vi "14_NOV_VARY_I_GET_V_FOR_LOOP.vi"() -> ()   [LabVIEW 2020]
uses:
  <instrlib>/Agilent B2900 Series/Agilent B2900 Series.lvlib
panel:
  out "SCPI COMMAND":string
  out "XY Graph":cluster{"X":dbl[], "Y":dbl[]}[](graph)
  out "Waveform Chart":dbl(graph)
  out "Measured Voltage (V)":dbl
  in  "SELECT DEVICE":refnum<visa-resource-name>="USB0::0x0957::0x8E18::MY51140695::INSTR"
  in  "Channel":enum16{"Not Selected", "1", "2"}(ring)
  out "Source Current (A)":dbl
  out "Resolution (A)":dbl format="%#_6f"
  in  "Specify number of steps":dbl
  in  "Set final Current(A)":dbl
  in  "Set initial Current(A)":dbl
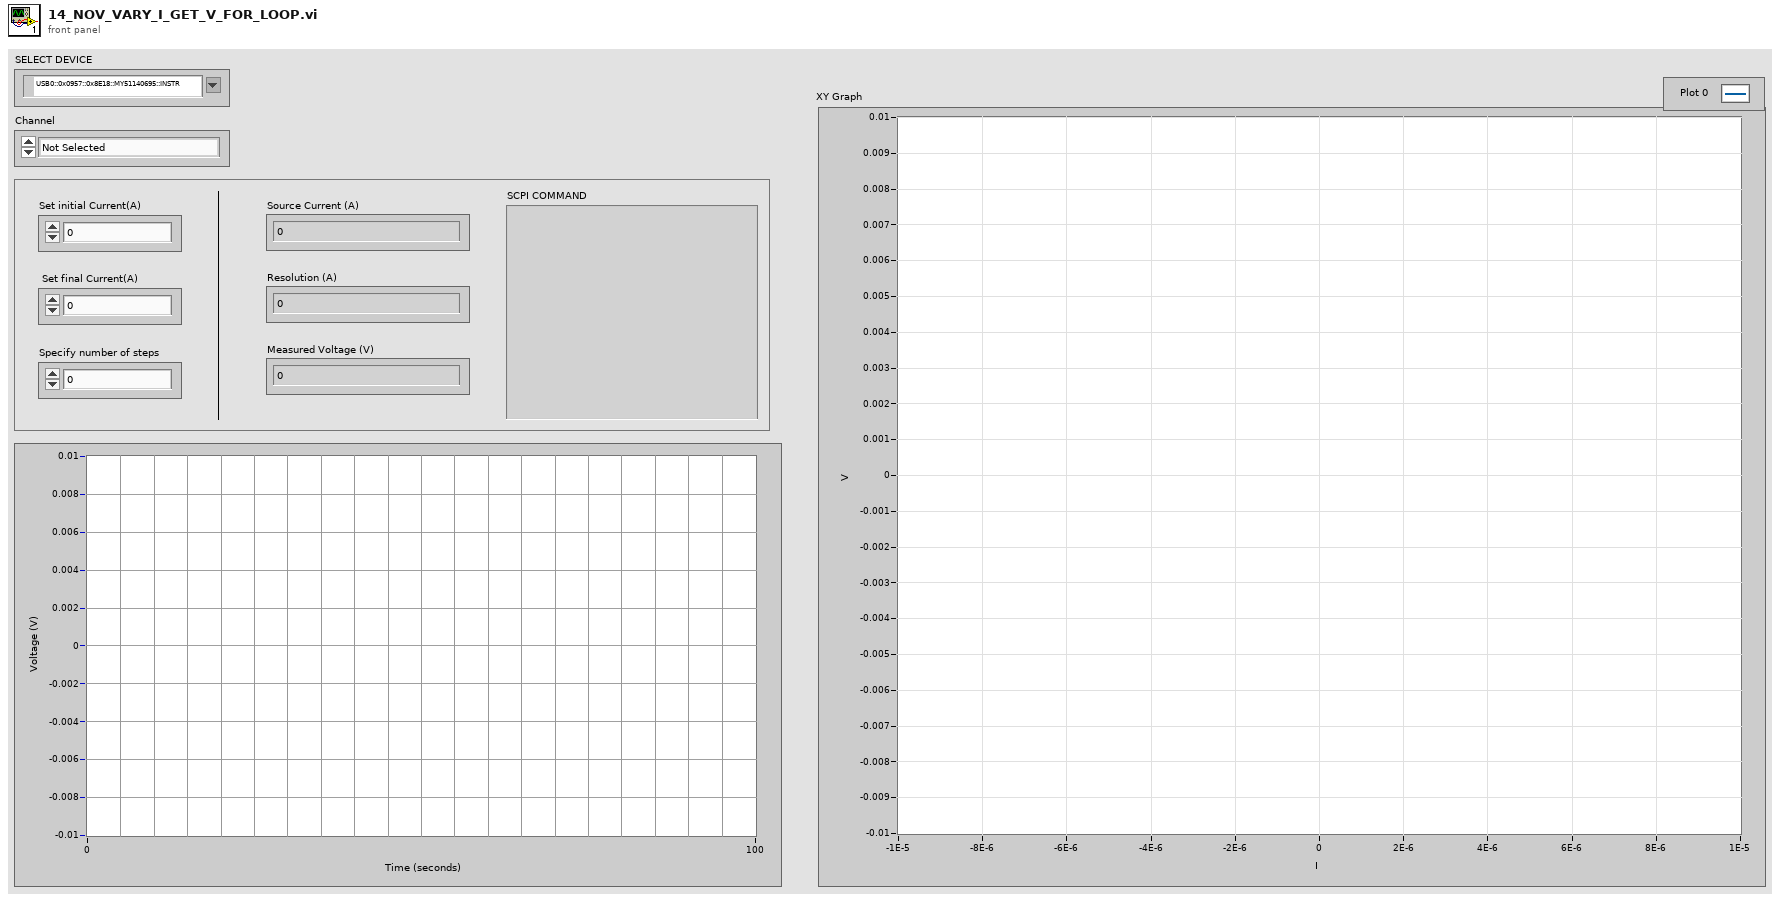
[diagram p1: front panel]
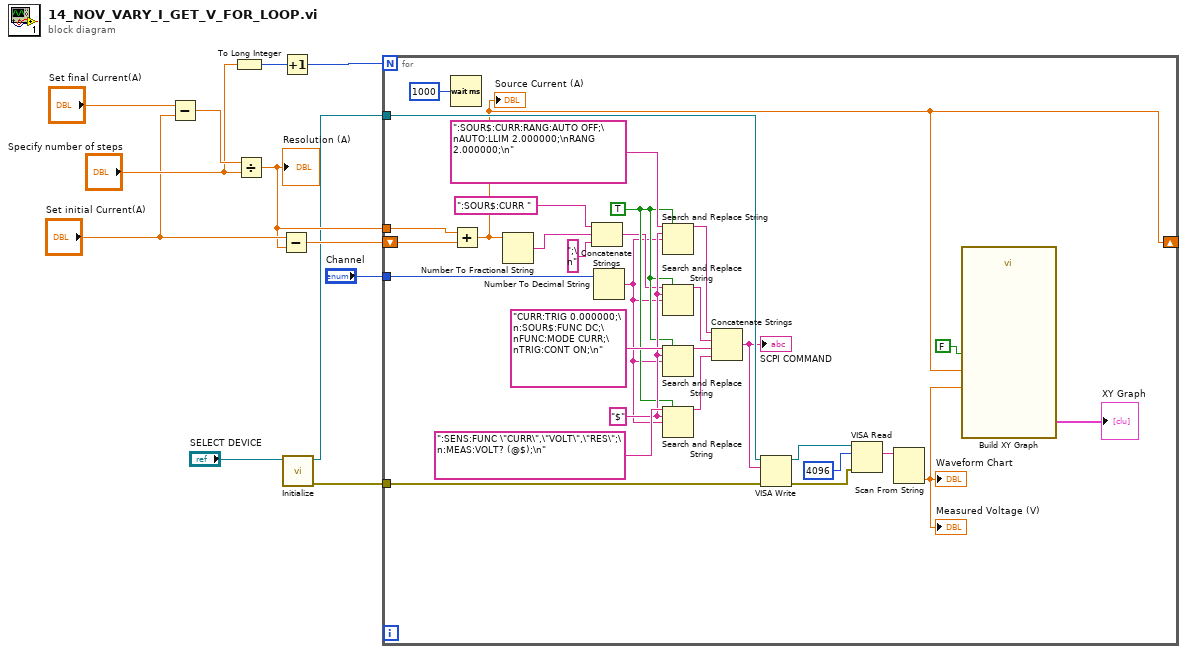
[diagram p0: block diagram]
diagram:
  n1 = Subtract(x="Set final Current(A)", y="Set initial Current(A)") -> (x-y=w11:dbl)
  n2 = To Long Integer(number="Specify number of steps") -> (32bit integer=w6:i32)
  n3 = Divide(x=w11, y="Specify number of steps") -> (x/y=w8:dbl)
  "Resolution (A)" <- w8
  n4 = Subtract(x="Set initial Current(A)", y=w8) -> (x-y=w7:dbl)
  n5 = Increment(x=w6) -> (x+1=w5:i32)
  n6 = call <instrlib>:"Initialize.vi"("VISA resource name"="SELECT DEVICE") -> ("error out"=w1:errorcluster, "VISA resource name out"=w2:refnum<visa-resource-name>)  [unwired: 9 in]
  n7 = for {
    N: w5 -> [_]
    shift-right: [w28] -> _
    shift-left: w7 -> [w41]
    tunnel: w8 -> [w40]
    tunnel: "Channel" -> [w38]
    tunnel: w2 -> [w33]
    tunnel: w1 -> [w32]
    w22 = "$" ("search string")
    w21 = TRUE ("replace all? (F)")
    n8 = Wait (ms)(milliseconds to wait=u32 1000) -> ()  [unwired: 1 out]
    n9 = Add(x=w40, y=w41) -> (x+y=w28:dbl)
    "Source Current (A)" <- w28
    n10 = Number To Fractional String(number=w28) -> (F-format string=w14:string)  [unwired: 3 in]
    n11 = Concatenate Strings(":SOUR$:CURR " ("string"), w14, ";\n" ("string")) -> (w16:string)
    n12 = Number To Decimal String(number=w38) -> (decimal integer string=w15:string)  [unwired: 1 in]
    n13 = Search and Replace String(replace all?=w21, input string=":SOUR$:CURR:RANG:AUTO OFF;\nAUTO:LLIM 2.000000;\nRANG 2.000000;\n", search string=w22, replace string=w15) -> (result string=w27:string)  [unwired: 4 in, 3 out]
    n14 = Search and Replace String(replace all?=w21, input string=w16, search string=w22, replace string=w15) -> (result string=w20:string)  [unwired: 4 in, 3 out]
    n15 = Search and Replace String(replace all?=w21, input string="CURR:TRIG 0.000000;\n:SOUR$:FUNC DC;\nFUNC:MODE CURR;\nTRIG:CONT ON;\n" ("string"), search string=w22, replace string=w15) -> (result string=w19:string)  [unwired: 4 in, 3 out]
    n16 = Search and Replace String(replace all?=w21, input string=":SENS:FUNC \"CURR\",\"VOLT\",\"RES\";\n:MEAS:VOLT? (@$);\n" ("string"), search string=w22, replace string=w15) -> (result string=w24:string)  [unwired: 4 in, 3 out]
    n17 = Concatenate Strings(w27, w20, w19, w24) -> (w13:string)
    "SCPI COMMAND" <- w13
    n18 = VISA Write(VISA resource name=w33, write buffer=w13, error in (no error)=w32) -> (VISA resource name out=w37:refnum<visa-resource-name>, error out=w36:errorcluster)  [unwired: 1 out]
    n19 = VISA Read(VISA resource name=w37, byte count=u32 4096, error in (no error)=w36) -> (read buffer=w34:string)  [unwired: 3 out]
    n20 = Scan From String(input string=w34) -> (output 1=w29:dbl)  [unwired: 4 in, 3 out]
    "Measured Voltage (V)" <- w29
    "Waveform Chart" <- w29
    n21 = call "Build XY Graph"("Reset"=FALSE, "Y Input"=w29, "X Input"=w28) -> ("XY Graph"=→"XY Graph":cluster{"X":dbl[], "Y":dbl[]}[])  [unwired: 7 in, 1 out]
  }
